vi "Stop Response.vi"(8 "error in (no error)":errorcluster, 10 "Name":string, 11 "Process Controller in":refnum<class "Process Controller.lvclass">) -> (0 "error out":errorcluster, 3 "Process Controller out":refnum<class "Process Controller.lvclass">)   [LabVIEW 2016, in "Process Controller.lvclass"]
uses:
  Process Controller.lvclass
  C:/github/LabActor/Worker/Worker.lvclass
  Process Controller.lvclass/Process Controller.ctl
  NHMFL_Core/Libraries/Instruments/Instrument Driver/Worker State.ctl
  Worker/Worker.lvclass/Worker.ctl
  Template Module/Write State.vi
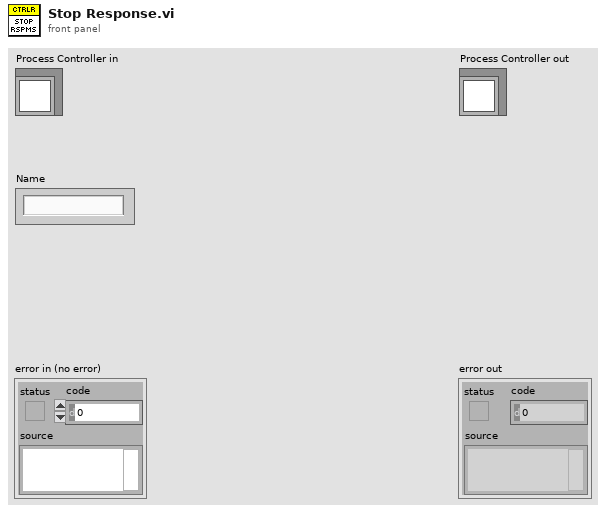
[diagram p1: front panel]
types:
  T1 = typedef "Worker State.ctl" = enum16{"Idle", "Starting", "Working", "Stopping"}
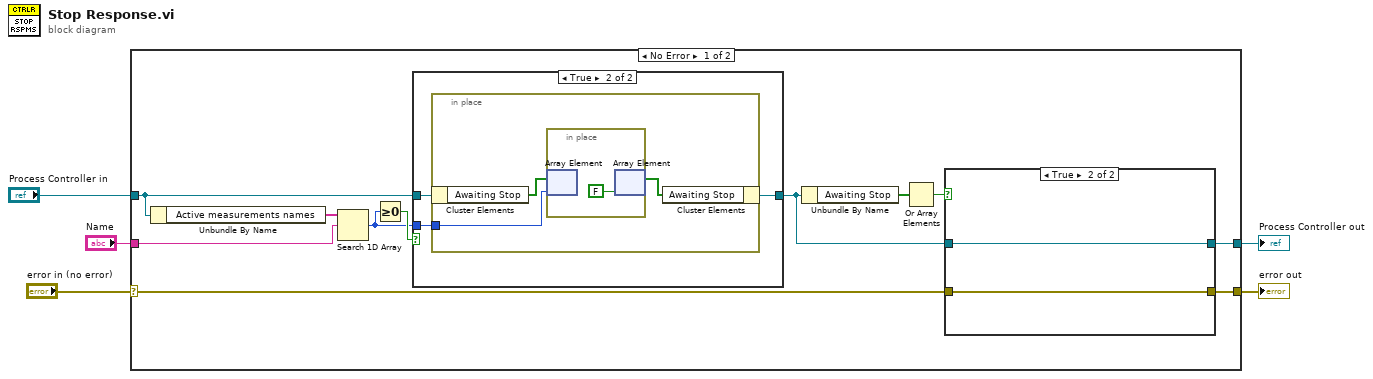
[diagram p0: block diagram]
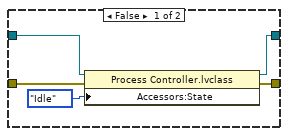
[diagram p2: hidden frame]
diagram:
  n1 = case shown="No Error" "error in (no error)" {
    selector: "error in (no error)" -> [w7 w33]
    tunnel: [w6 w33] -> w4
    tunnel: [w8 w32] -> w2
    tunnel: "Process Controller in" -> [w12 w32]
    tunnel: "Name" -> [w13 _]
    frame No Error {
      n2 = Unbundle By Name(w12) -> ("Active measurements names"=w16:string[])
      n3 = Search 1D Array(1D array=w16, element=w13) -> (index of element=w14:i32)  [unwired: 1 in]
      n4 = Greater Or Equal To 0?(x=w14) -> (x >= 0?=w15:bool)
      n5 = case shown="True" w15 {
        tunnel: w12 -> [w24 w27]
        tunnel: w14 -> [_ w26]
        tunnel: [w24 w25] -> w9
        frame False {
        }
        frame True {
          n6 = in-place {
            in-place-border: w26 -> [w28]
            n7 = in-place-cluster #1(w27) -> ("Awaiting Stop"=w30:bool[])
            n8 = in-place {
              n9 = in-place-array #2(w30, w28) -> ()  [unwired: 1 out]
              n10 = in-place-array #2(FALSE ("new element/subarray")) -> (w29:bool[])  [unwired: 1 out]
            }
            n11 = in-place-cluster #1("Awaiting Stop"=w29) -> (w25:refnum<class "Process Controller.lvclass">)
          }
        }
      }
      n12 = Unbundle By Name(w9) -> ("Awaiting Stop"=w11:bool[])
      n13 = Or Array Elements(Boolean array=w11) -> (logical OR=w10:bool)
      n14 = case shown="True" w10 {
        tunnel: w9 -> [w21 w23]
        tunnel: [w18 w23] -> w8
        tunnel: w7 -> [w20 w22]
        tunnel: [w19 w22] -> w6
        frame False {
          n15 = property class="Process Controller.lvclass"(reference=w21, error in=w20, "Accessors:State"=Worker_State."Idle" ("State")) -> (reference out=w18:refnum<class "Process Controller.lvclass">, error out=w19:errorcluster)
        }
        frame True {
        }
      }
    }
    frame Error {
    }
  }
  "error out" <- w4
  "Process Controller out" <- w2
